vi "Filter Menu Selection Event.vi"(8 "error in (no error)":errorcluster, 10 "MenuSelectionMsg":refnum<class "MenuSelectionMsg.lvclass">, 11 "IEventFilter in":refnum<class "IEventFilter.lvclass">) -> (0 "error out":errorcluster, 1 "Discard?":bool, 3 "IEventFilter out":refnum<class "IEventFilter.lvclass">)   [LabVIEW 2015, in "ActorEvents.lvlib" / "IEventFilter.lvclass"]
uses:
  IEventFilter.lvclass
  IEventAggregator Messages/MenuSelectionMsg/MenuSelectionMsg.lvclass
panel:
  # "No additional\nEvent Data"
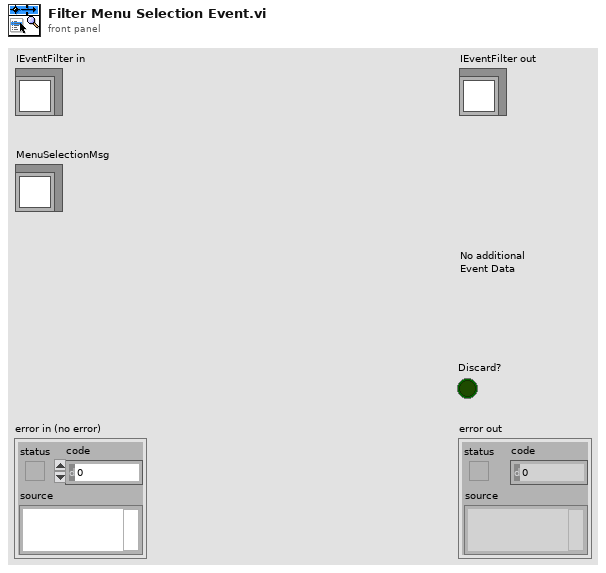
[diagram p1: front panel]
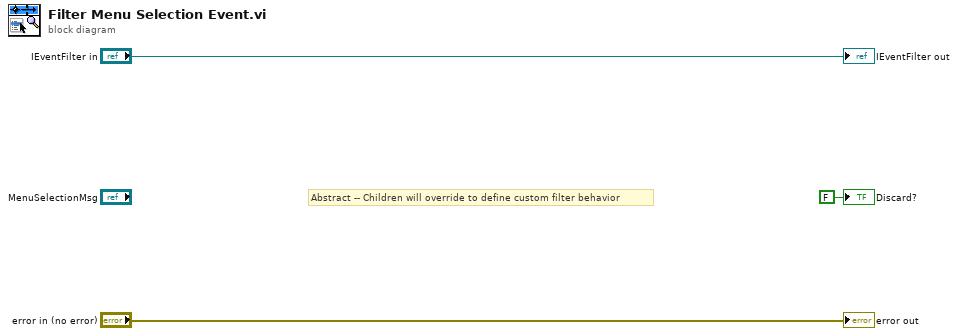
[diagram p0: block diagram]
diagram:
  # "Abstract -- Children will override to define custom filter behavior"
  "error out" <- "error in (no error)"
  "IEventFilter out" <- "IEventFilter in"
  "Discard?" <- FALSE ("Discard?")
